vi "Serialize.vi"(8 "error in (no error)":errorcluster, 10 "Element in":refnum<k20>, 11 "Test Suite in":refnum<class "Test Suite.lvclass">) -> (0 "error out":errorcluster, 2 "Element out":refnum<k20>)   [LabVIEW 2013, in "JUnit XML.lvlib" / "Test Suite.lvclass"]
doc: "Serializes a Test Suite using NI XML Parser."
uses:
  Test Suite.lvclass
  Test Case/Test Result.ctl
  Test Suite.lvclass/Test Suite.ctl
  <vilib>/xml/Close Reference(Node).vi
  JUnit XML.lvlib
  <vilib>/xml/NI_XML.lvlib
  Test Case/Test Case.lvclass
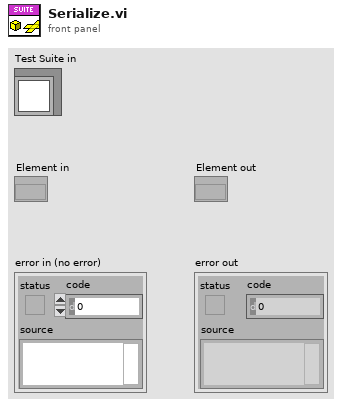
[diagram p1: front panel]
types:
  T1 = typedef "JUnit XML.lvlib/Test Case.lvclass/Test Result.ctl" = enum16{"Success", "Failure", "Error", "Skipped"}
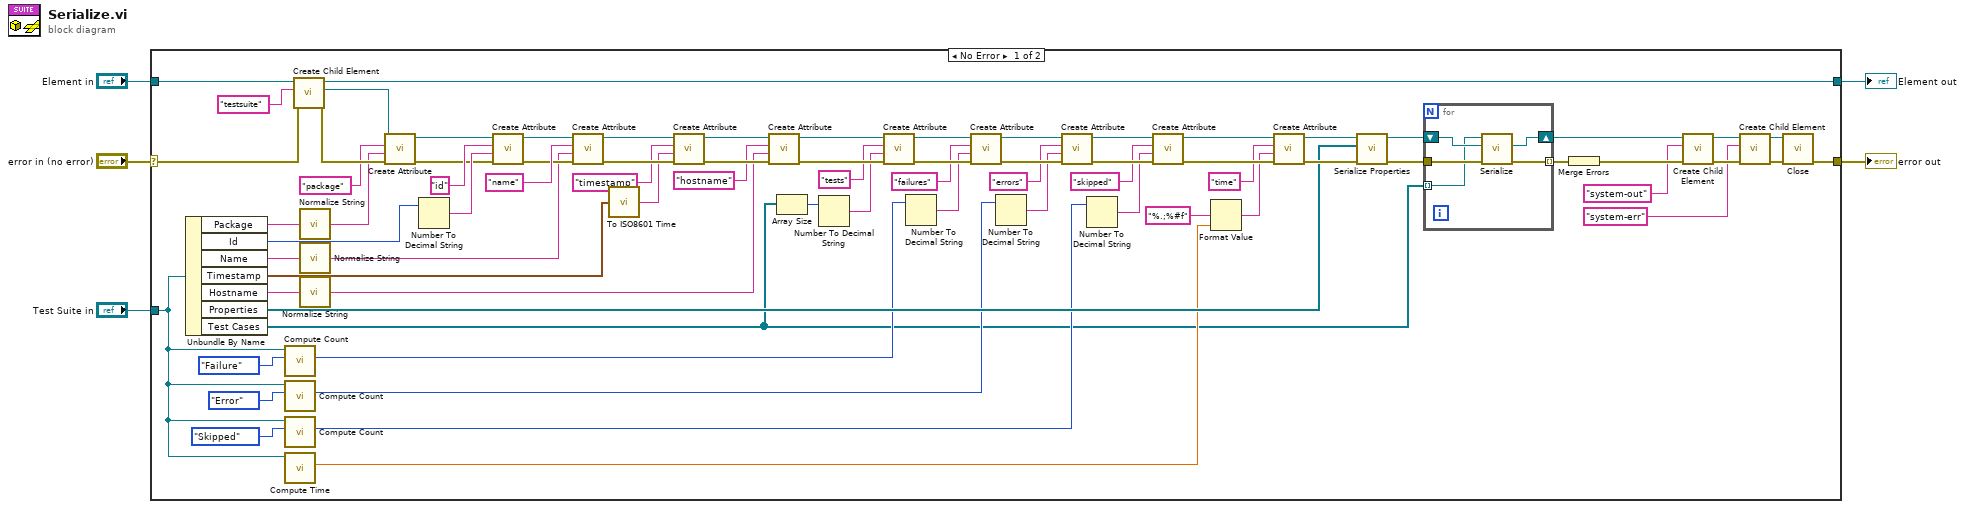
[diagram p0: block diagram]
diagram:
  n1 = case shown="No Error" "error in (no error)" {
    selector: "error in (no error)" -> [w36 w87]
    tunnel: [w21 w87] -> w4
    tunnel: "Test Suite in" -> [w13 _]
    tunnel: "Element in" -> [w35 w86]
    tunnel: [w34 w86] -> w1
    frame No Error {
      n2 = Unbundle By Name(w13) -> ("Package"=w37:string, "Id"=w44:i32, "Name"=w78:string, "Timestamp"=w74:timestamp, "Hostname"=w43:string, "Properties"=w20:refnum<class "Property.lvclass">[], "Test Cases"=w9:refnum<class "Test Case.lvclass">[])
      n3 = call "Compute Count.vi"("Test Result"=Test_Result."Failure", "Test Suite in"=w13) -> ("Count"=w11:i32)  [unwired: 7 in, 2 out]
      n4 = call "Compute Count.vi"("Test Result"=Test_Result."Error", "Test Suite in"=w13) -> ("Count"=w12:i32)  [unwired: 7 in, 2 out]
      n5 = call "Compute Count.vi"("Test Result"=Test_Result."Skipped", "Test Suite in"=w13) -> ("Count"=w17:i32)  [unwired: 7 in, 2 out]
      n6 = call "Compute Time.vi"("Test Suite in"=w13) -> ("Time"=w18:dbl)  [unwired: 8 in, 2 out]
      n7 = call "Create Child Element.vi"("error in (no error)"=w36, "Name"="testsuite" ("Tag Name"), "Element in"=w35) -> ("error out"=w41:errorcluster, "Child Element"=w40:refnum<k20>, "Element out"=w34:refnum<k20>)  [unwired: 6 in]
      n8 = call "Normalize String.vi"("String"=w37) -> ("Normalized String"=w8:string)  [unwired: 1 in]
      n9 = call "Normalize String.vi"("String"=w78) -> ("Normalized String"=w7:string)  [unwired: 1 in]
      n10 = call "Normalize String.vi"("String"=w43) -> ("Normalized String"=w6:string)  [unwired: 1 in]
      n11 = call "Create Attribute.vi"("error in (no error)"=w41, "Value"=w8, "Name"="package" ("Attribute Name"), "Element in"=w40) -> ("error out"=w42:errorcluster, "Element out"=w39:refnum<k20>)  [unwired: 6 in]
      n12 = Number To Decimal String(number=w44) -> (decimal integer string=w45:string)  [unwired: 1 in]
      n13 = call "Create Attribute.vi"("error in (no error)"=w42, "Value"=w45, "Name"="id" ("Attribute Name"), "Element in"=w39) -> ("error out"=w48:errorcluster, "Element out"=w47:refnum<k20>)  [unwired: 6 in]
      n14 = call "Create Attribute.vi"("error in (no error)"=w48, "Value"=w7, "Name"="name" ("Attribute Name"), "Element in"=w47) -> ("error out"=w76:errorcluster, "Element out"=w77:refnum<k20>)  [unwired: 6 in]
      n15 = call "To ISO8601 Time.vi"("Time Stamp"=w74) -> ("String"=w73:string)  [unwired: 1 in]
      n16 = call "Create Attribute.vi"("error in (no error)"=w76, "Value"=w73, "Name"="timestamp" ("Attribute Name"), "Element in"=w77) -> ("error out"=w71:errorcluster, "Element out"=w72:refnum<k20>)  [unwired: 6 in]
      n17 = call "Create Attribute.vi"("error in (no error)"=w71, "Value"=w6, "Name"="hostname" ("Attribute Name"), "Element in"=w72) -> ("error out"=w68:errorcluster, "Element out"=w69:refnum<k20>)  [unwired: 6 in]
      n18 = Array Size(array=w9) -> (size(s)=w10:i32)
      n19 = Number To Decimal String(number=w10) -> (decimal integer string=w66:string)  [unwired: 1 in]
      n20 = call "Create Attribute.vi"("error in (no error)"=w68, "Value"=w66, "Name"="tests" ("Attribute Name"), "Element in"=w69) -> ("error out"=w65:errorcluster, "Element out"=w64:refnum<k20>)  [unwired: 6 in]
      n21 = Number To Decimal String(number=w11) -> (decimal integer string=w62:string)  [unwired: 1 in]
      n22 = call "Create Attribute.vi"("error in (no error)"=w65, "Value"=w62, "Name"="failures" ("Attribute Name"), "Element in"=w64) -> ("error out"=w60:errorcluster, "Element out"=w61:refnum<k20>)  [unwired: 6 in]
      n23 = Number To Decimal String(number=w12) -> (decimal integer string=w58:string)  [unwired: 1 in]
      n24 = call "Create Attribute.vi"("error in (no error)"=w60, "Value"=w58, "Name"="errors" ("Attribute Name"), "Element in"=w61) -> ("error out"=w56:errorcluster, "Element out"=w57:refnum<k20>)  [unwired: 6 in]
      n25 = Number To Decimal String(number=w17) -> (decimal integer string=w54:string)  [unwired: 1 in]
      n26 = call "Create Attribute.vi"("error in (no error)"=w56, "Value"=w54, "Name"="skipped" ("Attribute Name"), "Element in"=w57) -> ("error out"=w52:errorcluster, "Element out"=w53:refnum<k20>)  [unwired: 6 in]
      n27 = Format Value(format string="%.;%#f", value (0)=w18) -> (output string=w49:string)  [unwired: 1 in]
      n28 = call "Create Attribute.vi"("error in (no error)"=w52, "Value"=w49, "Name"="time" ("Attribute Name"), "Element in"=w53) -> ("error out"=w22:errorcluster, "Element out"=w19:refnum<k20>)  [unwired: 6 in]
      n29 = call "Serialize Properties.vi"("error in (no error)"=w22, "Properties"=w20, "Node in"=w19) -> ("error out"=w31:errorcluster, "Node out"=w32:refnum<k20>)  [unwired: 7 in]
      n30 = for {
        tunnel: [w83] -> w33 mode=indexing
        tunnel: w31 -> [w82]
        shift-right: [w84] -> w30
        shift-left: w32 -> [w85]
        tunnel: w9 -> [w81] mode=indexing
        n31 = call "Serialize.vi"("error in (no error)"=w82, "Element in"=w85, "Test Case in"=w81) -> ("error out"=w83:errorcluster, "Element out"=w84:refnum<k20>)  [unwired: 7 in]
      }
      n32 = Merge Errors(w33) -> (w29:errorcluster)
      n33 = call "Create Child Element.vi"("error in (no error)"=w29, "Name"="system-out" ("Tag Name"), "Element in"=w30) -> ("error out"=w27:errorcluster, "Element out"=w28:refnum<k20>)  [unwired: 6 in, 1 out]
      n34 = call "Create Child Element.vi"("error in (no error)"=w27, "Name"="system-err" ("Tag Name"), "Element in"=w28) -> ("error out"=w26:errorcluster, "Element out"=w25:refnum<k20>)  [unwired: 6 in, 1 out]
      n35 = call-poly <vilib>:"Close.vi"("error in (no error)"=w26, "node"=w25) -> ("error out"=w21:errorcluster)  [unwired: 7 in]
    }
    frame Error {
    }
  }
  "error out" <- w4
  "Element out" <- w1
